vi "generate_square_plan.vi"(4 "error in (no error)":errorcluster, 5 "Accel length":dbl, 6 "Segments per side":i32, 7 "Radius":dbl) -> (0 "error out":errorcluster, 2 "Plan":string)   [LabVIEW 2020]
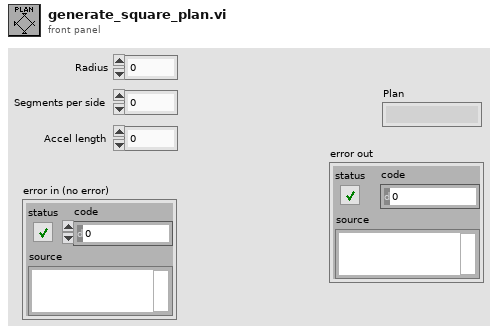
[diagram p1: front panel]
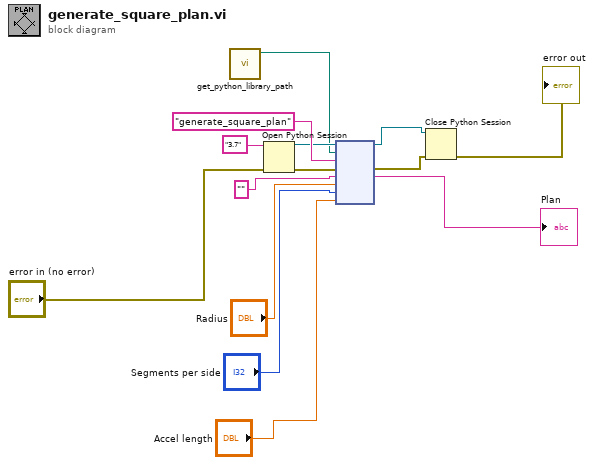
[diagram p0: block diagram]
diagram:
  n1 = call "get_python_library_path.vi"() -> ("Python library path"=w4:path)  [unwired: 11 in]
  n2 = Open Python Session(python version="3.7" ("Python version"), 3:"error in (no error)") -> (session out=w6:refnum<k35>, error out=w8:errorcluster)  [unwired: 1 in]
  n3 = node(w6, w4, "generate_square_plan" ("function name"), w8, "" ("Python version"), "Radius", "Segments per side", "Accel length") -> (w13:refnum<k35>, w14:errorcluster, →"Plan":string)  [unwired: 3 in, 2 out]
  n4 = Close Python Session(session in=w13, error in=w14) -> (11:→"error out":errorcluster)
